vi "GetScriptFromINIFile.vi"(8 "ErrorArray In":errorcluster[](array[cluster]), 11 "Path":path) -> (0 "ErrorArray Out":errorcluster[](array[cluster]), 3 "Script":string[](array[string]))   [LabVIEW 2014, in "TestFramework.lvlib"]
uses:
  TestFramework.lvlib
  <vilib>/Utility/error.llb/Error Cluster From Error Code.vi
  <vilib>/ErrorRing/Error Ring.xnode
  <vilib>/Utility/config.llb/NI_LVConfig.lvlib
  <userlib>/NIST/NISTErrorLib/NISTErrorLib.lvlib
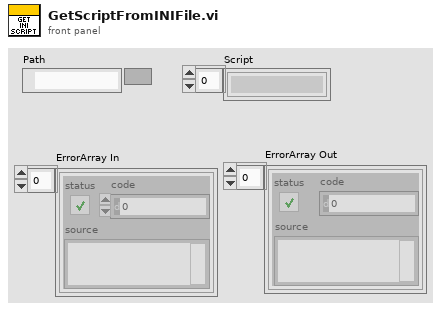
[diagram p1: front panel]
types:
  T1 = typedef "NI_LVConfig.lvlib/Config Data RefNum.ctl" = refnum<k1>
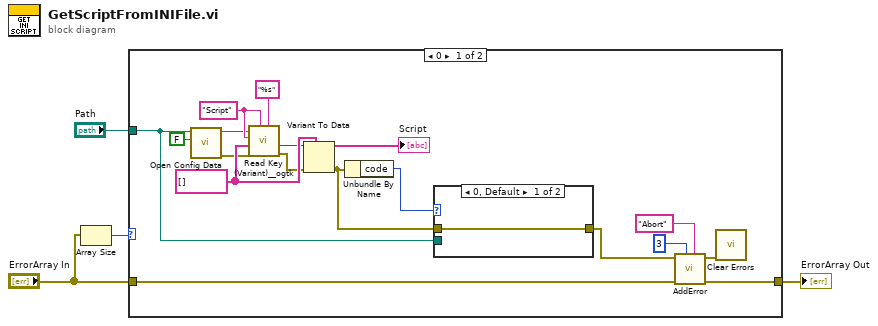
[diagram p0: block diagram]
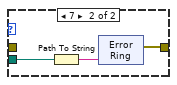
[diagram p2: hidden frame]
diagram:
  n1 = Array Size(array="ErrorArray In") -> (size(s)=w1:i32)
  n2 = case shown="0" w1 {
    tunnel: "Path" -> [w11 _]
    tunnel: [w6 w34] -> w3
    tunnel: "ErrorArray In" -> [w5 w34]
    frame 0 {
      w22 = string[] []
      w17 = "Script" ("section")
      n3 = call <vilib>:"Open Config Data.vi"("create file if necessary (T)"=FALSE, "configuration file path"=w11) -> ("error out"=w15:errorcluster, "refnum"=w16:T1)  [unwired: 7 in, 1 out]
      n4 = call <userlib>:"Read Key (Variant)__ogtk.vi"("format string (%;%f)"="%s", "section"=w17, "error in (no error)"=w15, "type"=w22, "key (optional)"=w17, "refnum"=w16) -> ("error out"=w21:errorcluster, "key-value"=w19:variant)  [unwired: 2 in, 2 out]
      n5 = Variant To Data(error in=w21, type=w22, Variant=w19) -> (data=→"Script":string[], error out=w12:errorcluster)
      n6 = Unbundle By Name(w12) -> ("code"=w13:i32)
      n7 = case shown="0, Default" w13 {
        tunnel: w12 -> [w23 _]
        tunnel: [w23 w24] -> w9
        tunnel: w11 -> [_ w25]
        frame 0, Default {
        }
        frame 7 {
          n8 = Path To String(path=w25) -> (string=w26:string)
          n9 = xnode "Error Ring"("parameter 0"=w26) -> ("error out"=w24:errorcluster)
        }
      }
      n10 = call <userlib>:"AddError.vi"("Severity"="Abort" ("String"), "Priority"=u8 3, "ErrorArray"=w5, "error in (no error)"=w9) -> ("ErrorArray"=w6:errorcluster[], "error out"=w10:errorcluster)  [unwired: 6 in]
      n11 = call <vilib>:"Clear Errors.vi"("error in (no error)"=w10) -> ()  [unwired: 5 in, 2 out]
    }
    frame 1, Default {
    }
  }
  "ErrorArray Out" <- w3
